vi "Set Single Track.vi"(8 "error in (no error)":errorcluster, 10 "height":i32, 11 "centre":i32) -> (0 "error out":errorcluster, 3 "function return":u32)   [LabVIEW 2014, in "atmcd32d.lvlib"]
doc: "unsigned int WINAPI SetSingleTrack(int centre, int height);"
uses:
  atmcd32d.lvlib
  atmcd32d.dll
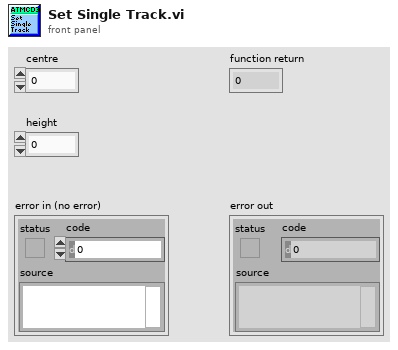
[diagram p1: front panel]
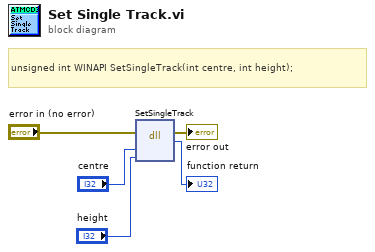
[diagram p0: block diagram]
diagram:
  # "unsigned int WINAPI SetSingleTrack(int centre, int height);"
  n1 = dll-call lib="C:/Users/Bakir/Documents/Lambda2-Testing/lib/Andorlib/atmcd32d.*" fn="SetSingleTrack"(error in="error in (no error)", "centre"="centre", "height"="height") -> (error out=→"error out":errorcluster, →"function return":u32)  [unwired: 4 in, 1 out]
